vi "Pack Transfer Parameters.vi"(8 "error in":errorcluster, 11 "Labeled Transfer Parameters":T3(array[cluster])) -> (0 "dup error out":errorcluster, 3 "Transfer Groups":T1[](array[typedef]))   [LabVIEW 2020, in "RDMA.lvlib" / "RDMA Transceiver.lvclass"]
doc: "Returns sorted transfer groups with sorted transfers within each group."
uses:
  RDMA Transceiver.lvclass
  DSF Core.lvlibp/Classes/Configuration/Core/Transfer/Transfer Configuration.lvclass
  Transfer Parameters.ctl
  Transfer Group Parameters.ctl
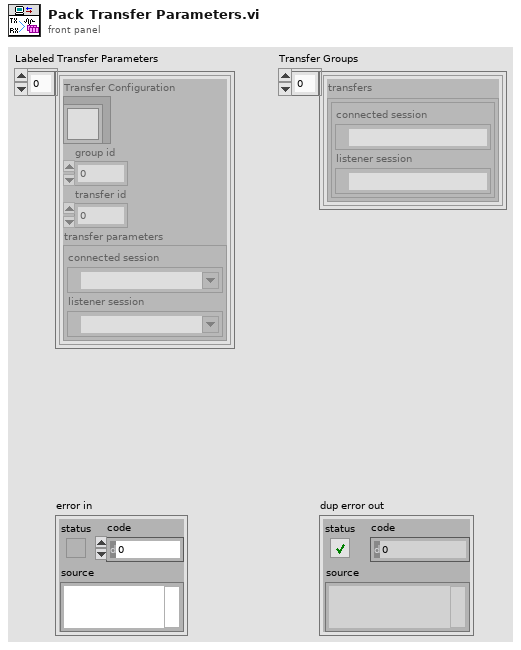
[diagram p1: front panel]
types:
  T1 = typedef "RDMA.lvlib/RDMA Transceiver.lvclass/Transfer Group Parameters.ctl" = cluster{"transfers":T2[]}
  T2 = typedef "RDMA.lvlib/RDMA Transceiver.lvclass/Transfer Parameters.ctl" = cluster{"connected session":refnum<k21>, "listener session":refnum<k21>}
  T3 = cluster{"Transfer Configuration":refnum<class "Transfer Configuration.lvclass">, "group id":i32, "transfer id":i32, "transfer parameters":T2}[]
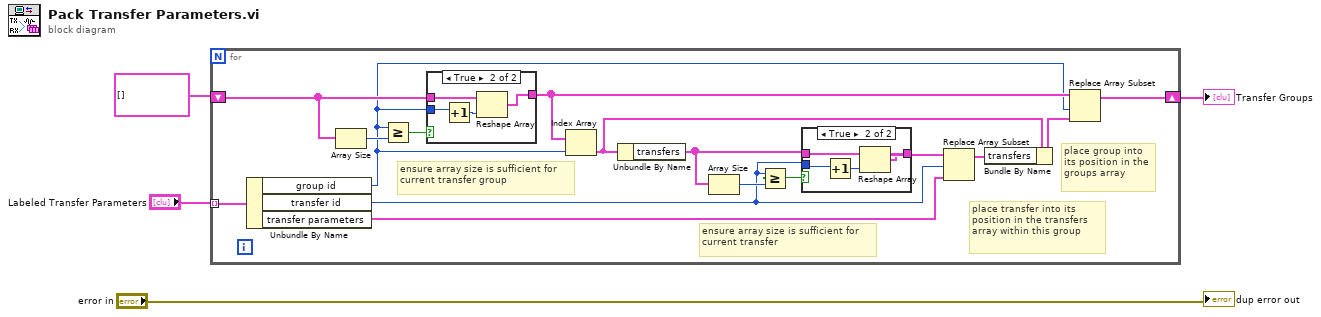
[diagram p0: block diagram]
diagram:
  n1 = for {
    shift-right: [w14] -> w2
    shift-left: T1[] [] ("initialized array") -> [w11]
    tunnel: "Labeled Transfer Parameters" -> [w8] mode=indexing
    # "place group into its position in the groups array"
    # "place transfer into its position in the transfers array within this group"
    # "ensure array size is sufficient for current transfer"
    # "ensure array size is sufficient for current transfer group"
    n2 = Unbundle By Name(w8) -> ("group id"=w5:i32, "transfer id"=w6:i32, "transfer parameters"=w7:T2)
    n3 = Array Size(array=w11) -> (size(s)=w9:i32)
    n4 = Greater Or Equal?(x=w5, y=w9) -> (x >= y?=w12:bool)
    n5 = case shown="True" w12 {
      tunnel: [w21 w22] -> w10
      tunnel: w11 -> [w21 w24]
      tunnel: w5 -> [_ w23]
      frame False {
      }
      frame True {
        n6 = Increment(x=w23) -> (x+1=w25:i32)
        n7 = Reshape Array(w24, w25) -> (w22:T1[])
      }
    }
    n8 = Index Array(array=w10, index=w5) -> (element=w17:T1)
    n9 = Unbundle By Name(w17) -> ("transfers"=w18:T2[])
    n10 = Array Size(array=w18) -> (size(s)=w13:i32)
    n11 = Greater Or Equal?(x=w6, y=w13) -> (x >= y?=w19:bool)
    n12 = case shown="True" w19 {
      tunnel: w18 -> [w26 w30]
      tunnel: w6 -> [_ w29]
      tunnel: [w26 w28] -> w20
      frame False {
      }
      frame True {
        n13 = Increment(x=w29) -> (x+1=w27:i32)
        n14 = Reshape Array(w30, w27) -> (w28:T2[])
      }
    }
    n15 = Replace Array Subset(array=w20, new element=w7, index=w6) -> (w16:T2[])
    n16 = Bundle By Name(cluster=w17, "transfers"=w16) -> (w15:T1)
    n17 = Replace Array Subset(array=w10, new element=w15, index=w5) -> (w14:T1[])
  }
  "Transfer Groups" <- w2
  "dup error out" <- "error in"
